vi "Step-By-Step Tab Window.vi"(8 "error in (no error)":errorcluster) -> (0 "error out":errorcluster, 1 "Cancel?":bool)   [LabVIEW 2017]
panel:
  in  "OK":bool
  in  "Next":bool
  in  "Previous":bool
  in  "Tab Control":enum32{"Page 1", "Page 2", "Page 3", "Page 4"}(tab)
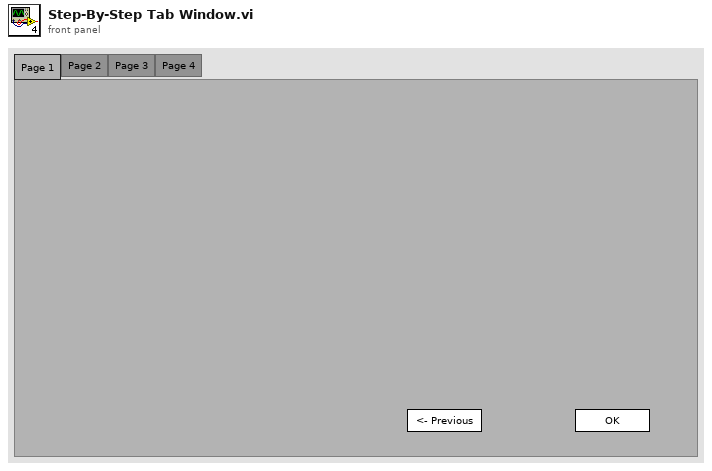
[diagram p1: front panel]
types:
  T1 = cluster{"TabControl":refnum<vi>, "Prev":refnum<vi>, "Next":refnum<vi>, "Finish":refnum<vi>}
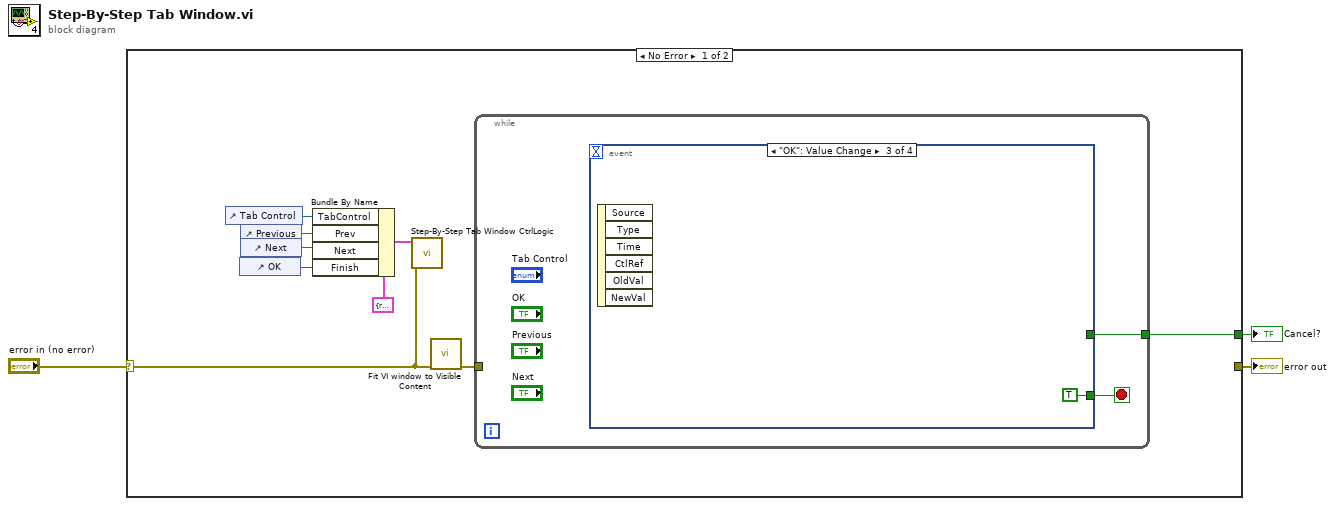
[diagram p0: block diagram]
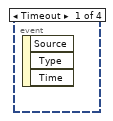
[diagram p2: hidden frame]
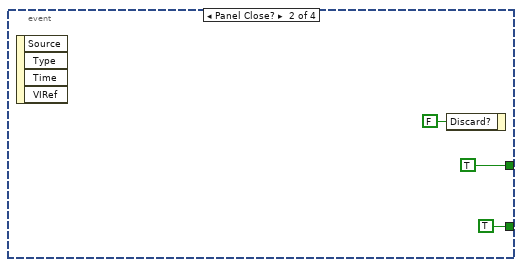
[diagram p3: hidden frame]
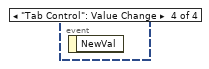
[diagram p4: hidden frame]
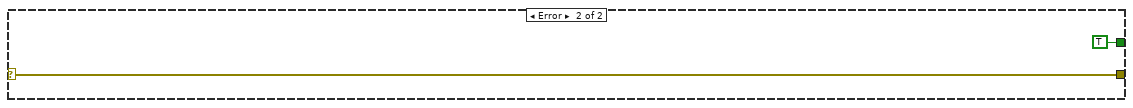
[diagram p5: hidden frame]
diagram:
  n1 = case shown="No Error" "error in (no error)" {
    selector: "error in (no error)" -> [w6 w20]
    tunnel: [_ w20] -> w2
    tunnel: [w5 TRUE] -> w1
    frame No Error {
      n2 = control-ref of="Tab Control"() -> (w10:refnum<vi>)
      n3 = control-ref of="OK"() -> (w7:refnum<vi>)
      n4 = control-ref of="Previous"() -> (w9:refnum<vi>)
      n5 = control-ref of="Next"() -> (w8:refnum<vi>)
      n6 = Bundle By Name(cluster=T1 {"TabControl"=refnum, "Prev"=refnum, "Next"=refnum, "Finish"=refnum} ("CtrlRef"), "TabControl"=w10, "Prev"=w9, "Next"=w8, "Finish"=w7) -> (w11:T1)
      n7 = call "Step-By-Step Tab Window CtrlLogic.vi"("error in (no error)"=w6, "CtrlRef"=w11) -> ()  [unwired: 10 in]
      n8 = call "Fit VI window to Visible Content.vi"("error in (no error)"=w6) -> ("error out"=w4:errorcluster)  [unwired: 5 in, 1 out]
      n9 = while {
        tunnel: w4 -> [_]
        tunnel: [w13] -> w5
        stop <- w14 stop-if-true
        n10 = event shown="[2] \"OK\": Value Change" {
          selector: _ -> [_ _ _ _]
          dyn-events: _ -> [_ _ _ _]
          timeout: _ -> [_ _ _ _]
          tunnel: [_ TRUE ("Discard?") TRUE ("Discard?") _] -> w14
          tunnel: [_ TRUE _ _] -> w13
          event Timeout {
            n11 = event-data() -> ()  [unwired: 1 in, 3 out]
          }
          event Panel Close? {
            n12 = event-data() -> ()  [unwired: 1 in, 4 out]
            n13 = event-data("Discard?"=FALSE) -> ()  [unwired: 1 in, 1 out]
          }
          event "OK": Value Change {
            n14 = event-data() -> ()  [unwired: 1 in, 6 out]
          }
          event "Tab Control": Value Change {
            n15 = event-data() -> ()  [unwired: 1 in, 1 out]
          }
        }
      }
    }
    frame Error {
    }
  }
  "error out" <- w2
  "Cancel?" <- w1
